vi "主函数.vi"() -> ()   [LabVIEW 2020]
doc: "UDP协议与TCP的区别在于UDP不包括发送数据包信息的错误检查，因此无法保证接收端是否已接收所发数据。\n\nUDP可用于“广播”数据至整个网络，只需指定可包括全部的IP地址(255.255.255.255)以便发送信息至整个网络。 由于路由器或其他网络硬件通常拒绝转发超过一定点的数据，在实际应用中广播范围可能存在限制。"
panel:
  in  "输出文件夹名称":path
  out "当前采集数据IP地址":string
  out "数据状态":string
  in  "数据采集卡IP地址":string
  out "输出波形":waveform(i32)[](graph)
  in  "停止 2":bool
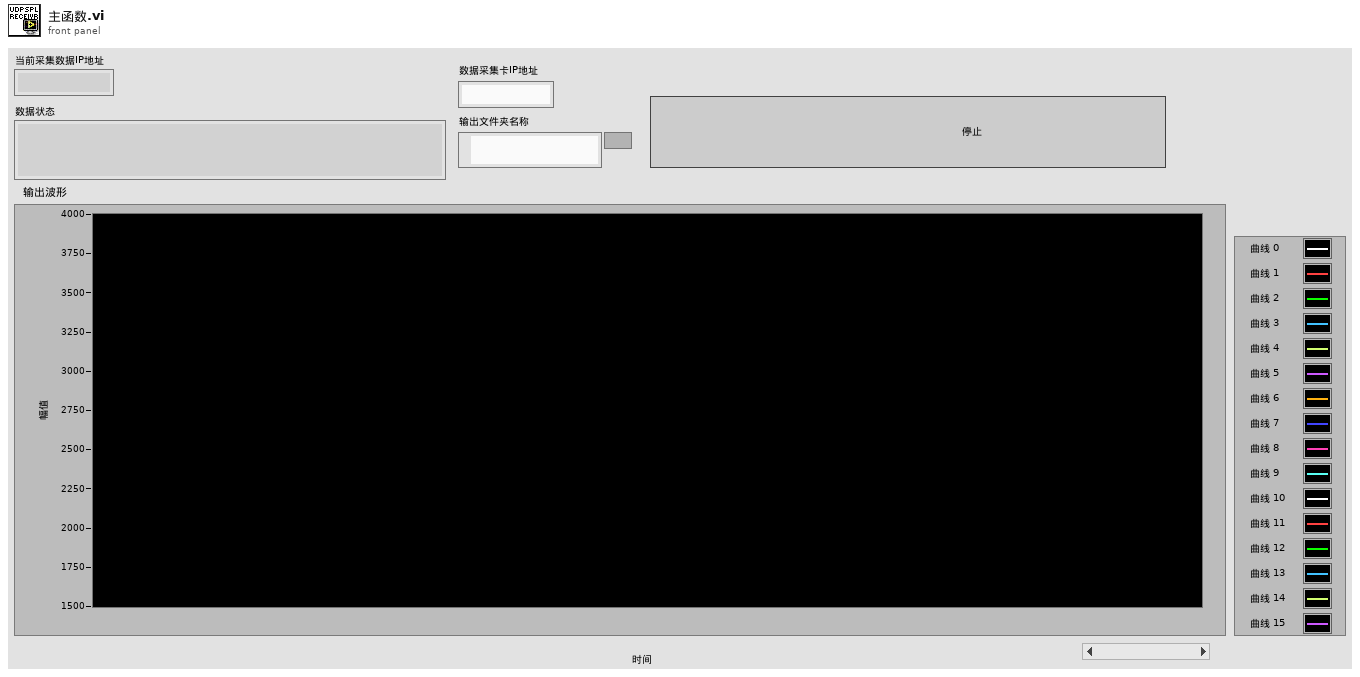
[diagram p1: front panel]
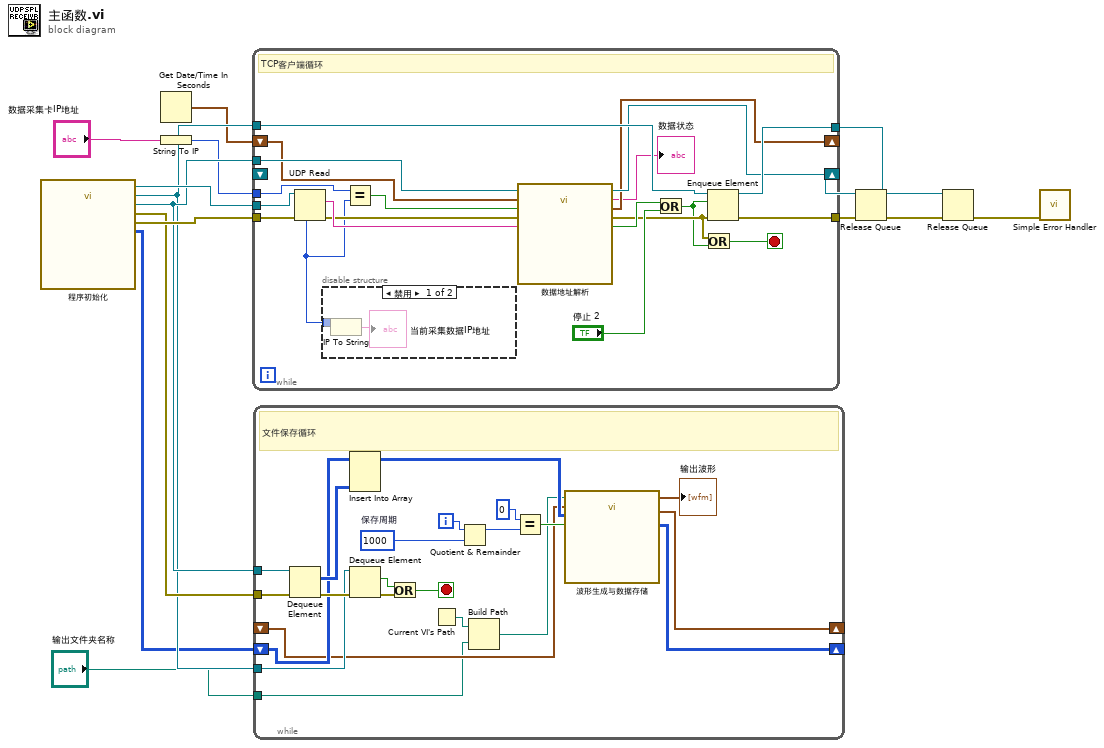
[diagram p0: block diagram]
diagram:
  n1 = call "程序初始化.vi"() -> ("错误输出"=w10:errorcluster, "queue out 2"=w9:refnum<queue>, "queue out"=w8:refnum<queue>, "UDP网络连接输出"=w15:refnum<k16>, "error out 2"=w14:errorcluster, "数组"=w6:i32[][])  [unwired: 6 in]
  n2 = Get Date/Time In Seconds() -> (seconds since 1Jan1904=w3:timestamp)
  n3 = String To IP(1:"数据采集卡IP地址") -> (0:w4:u32)
  n4 = while {
    tunnel: w14 -> [w33]
    tunnel: w15 -> [w32]
    tunnel: w8 -> [w31]
    tunnel: [w30] -> w11
    tunnel: w9 -> [w28]
    shift-right: [w29] -> w7
    shift-left: _ -> [_]
    tunnel: w4 -> [w27]
    shift-right: [w18] -> _
    shift-left: w3 -> [w25]
    tunnel: [w20] -> w2
    stop <- w35 stop-if-true
    # "TCP客户端循环"
    n5 = UDP Read(connection ID=w32, 8:w33) -> (data out=w34:string, error out=w22:errorcluster, 6:w16:u32)  [unwired: 1 in, 3 out]
    n6 = disable-structure shown="禁用" {
      disable-tunnel: w16 -> [w37 _]
      frame Disabled {
        n7 = IP To String(2:w37) -> (0:→"当前采集数据IP地址":string)  [unwired: 1 in]
      }
      frame Enabled {
      }
    }
    n8 = Equal?(x=w27, y=w16) -> (x = y?=w26:bool)
    n9 = call "数据地址解析.vi"("输入数据"=w34, "错误输入（无错误）"=w22, "地址判断位"=w26, "上轮成功输入时间"=w25, "回传数据队列"=w28) -> ("错误输出"=w21:errorcluster, "输出时间"=w18:timestamp, "数据状态"=→"数据状态":string, "回传数据队列"=w29:refnum<queue>, "超时标志位"=w23:bool)  [unwired: 2 in]
    n10 = Or(x=w23, y="停止 2") -> (x .or. y?=w19:bool)
    n11 = Or(x=w21, y=w19) -> (x .or. y?=w35:bool)
    n12 = Enqueue Element(queue=w31, element=w19, error in (no error)=w21) -> (queue out=w30:refnum<queue>, error out=w20:errorcluster)  [unwired: 1 in, 1 out]
  }
  n13 = while {
    tunnel: w10 -> [w59]
    tunnel: w9 -> [w57]
    tunnel: w8 -> [w55]
    shift-right: [w44] -> _
    shift-left: w6 -> [w51]
    shift-right: [w43] -> _
    shift-left: _ -> [w42]
    tunnel: "输出文件夹名称" -> [w38]
    i -> [w50]
    stop <- w58 stop-if-true
    w49 = 1000  # 保存周期
    # "文件保存循环"
    n14 = Dequeue Element(queue=w57, error in (no error)=w59) -> (element=w52:i32[][], error out=w56:errorcluster)  [unwired: 1 in, 2 out]
    n15 = Insert Into Array(array=w51, new element=w52) -> (w45:i32[][])  [unwired: 2 in]
    n16 = Dequeue Element(queue=w55, error in (no error)=w56) -> (element=w54:bool, error out=w53:errorcluster)  [unwired: 1 in, 2 out]
    n17 = Or(x=w54, y=w53) -> (x .or. y?=w58:bool)
    n18 = Current VI's Path() -> (path=w41:path)
    n19 = Quotient & Remainder(x=w50, y=w49) -> (x-y*floor(x/y)=w47:i32)  [unwired: 1 out]
    n20 = Build Path(base path=w41, name or relative path=w38) -> (appended path=w40:path)
    n21 = Equal?(x=0, y=w47) -> (x = y?=w46:bool)
    n22 = call "波形生成与数据存储.vi"("文件保存控制位"=w46, "数据输入"=w45, "上一时刻时间输入"=w42, "文件存储地址"=w40) -> ("缓存区输出"=w44:i32[][], "时间输出"=w43:timestamp, "波形图表 6"=→"输出波形":waveform(i32)[])  [unwired: 5 in]
  }
  n23 = Release Queue(queue=w7, error in (no error)=w2) -> (error out=w13:errorcluster)  [unwired: 1 in, 2 out]
  n24 = Release Queue(queue=w11, error in (no error)=w13) -> (error out=w12:errorcluster)  [unwired: 1 in, 2 out]
  n25 = call <vilib>:"Simple Error Handler.vi"("error in (no error)"=w12) -> ()  [unwired: 4 in, 5 out]
